vi "Untitled 1.vi"() -> ()   [LabVIEW 2020]
uses:
  <vilib>/Instr/_visa.llb/VISA Configure Serial Port (Instr).vi
panel:
  in  "Select COM Port":refnum<visa-resource-name>
  in  "LED 4":bool
  in  "LED 3":bool
  in  "LED 2":bool
  in  "LED 1":bool
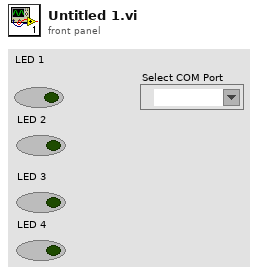
[diagram p1: front panel]
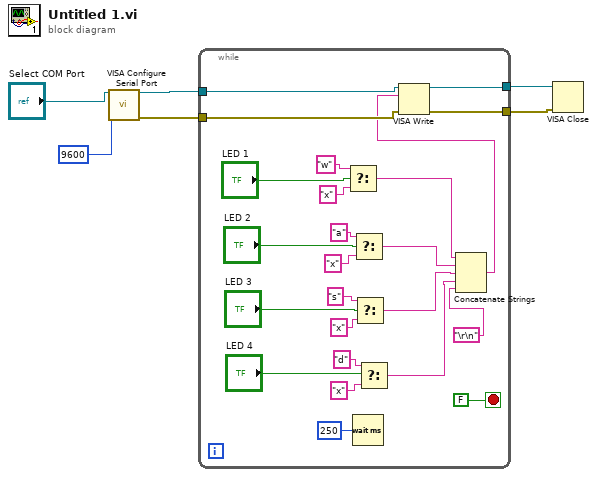
[diagram p0: block diagram]
diagram:
  n1 = call-poly "VISA Configure Serial Port"("VISA resource name"="Select COM Port", "baud rate (9600)"=u32 9600) -> ("VISA resource name out"=w4:refnum<visa-resource-name>, "error out"=w3:errorcluster)  [unwired: 12 in]
  n2 = while {
    tunnel: w4 -> [w11]
    tunnel: w3 -> [w10]
    tunnel: [w8] -> w1
    tunnel: [w7] -> w2
    stop <- FALSE stop-if-true
    n3 = Select(t="w", s="LED 1", f="x") -> (s? t:f=w18:string)
    n4 = Wait (ms)(milliseconds to wait=u32 250) -> ()  [unwired: 1 out]
    n5 = Select(t="a", s="LED 2", f="x") -> (s? t:f=w17:string)
    n6 = Select(t="s", s="LED 3", f="x") -> (s? t:f=w16:string)
    n7 = Select(t="d", s="LED 4", f="x") -> (s? t:f=w15:string)
    n8 = Concatenate Strings(w18, w17, w16, w15, "\r\n") -> (w9:string)
    n9 = VISA Write(VISA resource name=w11, write buffer=w9, error in (no error)=w10) -> (VISA resource name out=w7:refnum<visa-resource-name>, error out=w8:errorcluster)  [unwired: 1 out]
  }
  n10 = VISA Close(VISA resource name=w2, error in (no error)=w1) -> ()  [unwired: 1 out]
